vi "题目2.vi"() -> ()   [LabVIEW 2017]
panel:
  out "和2":dbl
  out "和1":dbl
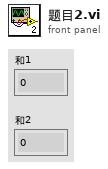
[diagram p1: front panel]
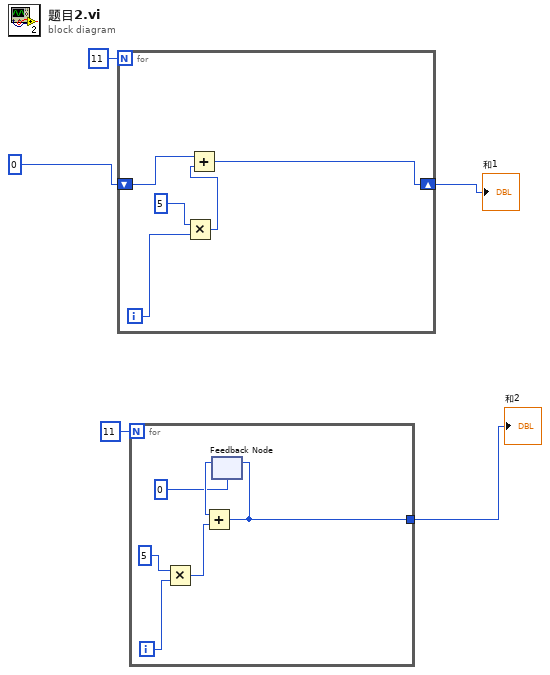
[diagram p0: block diagram]
diagram:
  n1 = for {
    N: 11 -> [_]
    shift-right: [w7] -> w4
    shift-left: 0 -> [w6]
    i -> [w8]
    n2 = Multiply(x=5, y=w8) -> (x*y=w10:i32)
    n3 = Add(x=w6, y=w10) -> (x+y=w7:i32)
  }
  "和1" <- w4
  n4 = for {
    N: 11 -> [_]
    tunnel: [w12] -> w1
    i -> [w16]
    n5 = Multiply(x=5, y=w16) -> (x*y=w14:i32)
    n6 = feedback #1(0) -> (w13:i32)
    n7 = Add(x=w13, y=w14) -> (x+y=w12:i32)
    n8 = feedback-in #1(w12) -> ()
  }
  "和2" <- w1
